vi "Ask Are you the Bearer.vi"(8 "error in (no error)":errorcluster, 10 "Guardian ID":string, 11 "Guardian in":refnum<class "Guardian.lvclass">) -> (0 "error out":errorcluster, 2 "Yes":bool, 3 "Guardian out":refnum<class "Guardian.lvclass">)   [LabVIEW 2026, in "TALOS.lvlib" / "Guardian.lvlib" / "Guardian.lvclass"]
uses:
  Guardian.lvclass
  TALOS.lvlib
  Classes/Guardian List/Guardian List.lvclass
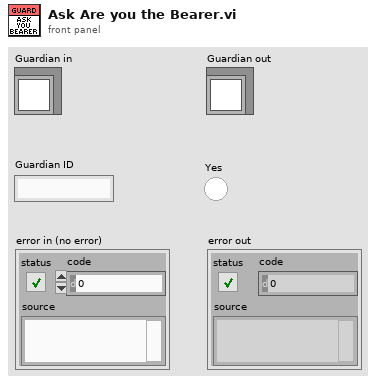
[diagram p1: front panel]
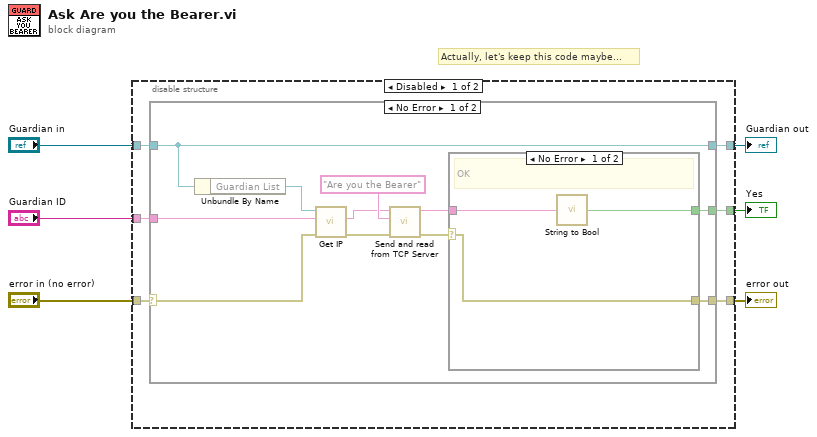
[diagram p0: block diagram]
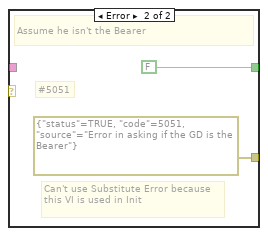
[diagram p2: hidden frame]
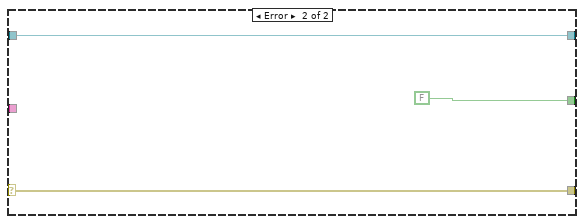
[diagram p3: hidden frame]
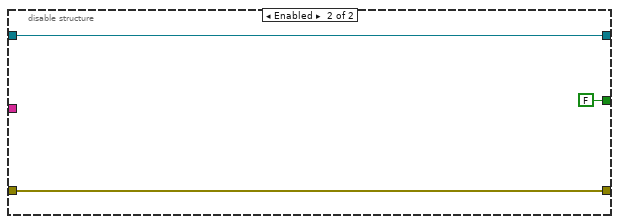
[diagram p4: hidden frame]
diagram:
  # "Actually, let's keep this code maybe..."
  n1 = disable-structure shown="Disabled" {
    disable-tunnel: "Guardian in" -> [w12 w32]
    disable-tunnel: "error in (no error)" -> [w11 w34]
    disable-tunnel: "Guardian ID" -> [w10 _]
    disable-tunnel: [w9 w32] -> w3
    disable-tunnel: [w8 FALSE ("Yes")] -> w2
    disable-tunnel: [w7 w34] -> w1
    frame Disabled {
      n2 = case shown="No Error" w11 {
        selector: w11 -> [w20 w29]
        tunnel: w12 -> [w16 w31]
        tunnel: w10 -> [w21 _]
        tunnel: [w16 w31] -> w9
        tunnel: [w14 FALSE] -> w8
        tunnel: [w13 w29] -> w7
        frame No Error {
          n3 = Unbundle By Name(w16) -> ("Guardian List"=w22:refnum<class "Guardian List.lvclass">)
          n4 = call-dynamic "Get IP.vi"("error in (no error)"=w20, "ID"=w21, "Guardian List in"=w22) -> ("error out"=w19:errorcluster, "IP"=w18:string)  [unwired: 6 in, 1 out]
          n5 = call "Send and read from TCP Server.vi"("error in (no error)"=w19, "Message"="Are you the Bearer", "GD ID"=w18) -> ("error out"=w15:errorcluster, "Reply"=w17:string)  [unwired: 7 in]
          n6 = case shown="No Error" w15 {
            selector: w15 -> [w24 _]
            tunnel: w17 -> [w26 _]
            tunnel: [w25 FALSE ("Boolean")] -> w14
            tunnel: [w24 errorcluster {"status"=TRUE, "code"=5051, "source"="Error in asking if the GD is the Bearer"} ("error IO")] -> w13
            frame No Error {
              # "OK"
              n7 = call "String to Bool.vi"("String"=w26) -> ("Boolean"=w25:bool)
            }
            frame Error {
              # "#5051"
              # "Can't use Substitute Error because this VI is used in Init"
              # "Assume he isn't the Bearer"
            }
          }
        }
        frame Error {
        }
      }
    }
    frame Enabled {
    }
  }
  "error out" <- w1
  "Guardian out" <- w3
  "Yes" <- w2
